vi "Process.vi"(8 "error in":errorcluster, 11 "Plugin in":refnum<class "StreamReader.lvclass">) -> (0 "error out":errorcluster, 3 "Plugin out":refnum<class "StreamReader.lvclass">)   [LabVIEW 2024, in "StreamReader.lvlib" / "StreamReader.lvclass"]
uses:
  StreamReader.lvclass
  C:/Program Files/National Instruments/LabVIEW 2024/vi.lib/FlexLogger/SDK/PluginSDK.lvlibp/PEFClasses/SDK/Plugin/Plugin.lvclass
  StreamReader.lvclass/StreamReader.ctl
  <vilib>/FlexLogger/SDK/PluginSDK.lvlibp/PEFClasses/SDK/Plugin/DataHelpers/Write 1D Wfm (DBL)_v2.vi
  <vilib>/FlexLogger/SDK/PluginSDK.lvlibp/PEFClasses/SDK/Plugin/Plugin.lvclass
  C:/Program Files/National Instruments/LabVIEW 2024/vi.lib/FlexLogger/SDK/PluginSDK.lvlibp/PEFClasses/SDK/Processing Element/Processing Element.lvclass
  C:/Users/Administrator/Documents/LabVIEW Projects/FlexLogger IO Plug-ins/StreamReader/StreamReader.lvclass
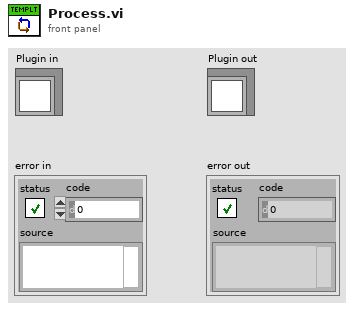
[diagram p1: front panel]
types:
  T1 = typedef "StreamReader.lvlib/StreamReader.lvclass/StreamReader Parameters.ctl" = cluster{"Reader URL":string, "Writer URL":string, "Timeout":i32, "Buffer Size":i32, "Reader endpoint":refnum<k21>, "Channel Names":string[]}
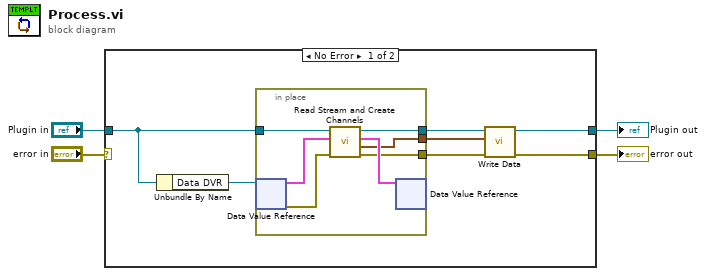
[diagram p0: block diagram]
diagram:
  n1 = case shown="No Error" "error in" {
    selector: "error in" -> [_ w19]
    tunnel: [w10 w20] -> w1
    tunnel: "Plugin in" -> [w5 w20]
    tunnel: [w11 w19] -> w2
    frame No Error {
      n2 = Unbundle By Name(w5) -> ("Data DVR"=w9:refnum<data-value>)
      n3 = in-place {
        in-place-border: w5 -> [w18]
        in-place-border: [w15] -> w8
        in-place-border: [w13] -> w7
        in-place-border: [w12] -> w6
        n4 = in-place-dvr #1(w9) -> (w17:T1, w16:errorcluster)
        n5 = call-dynamic "Read Stream and Create Channels.vi"("error in (no error)"=w16, "StreamReader Parameters in"=w17, "Plugin in"=w18) -> ("error out"=w13:errorcluster, "Array"=w12:waveform(dbl)[], "StreamReader Parameters out"=w14:T1, "Plugin out"=w15:refnum<class "StreamReader.lvclass">)  [unwired: 5 in]
        n6 = in-place-dvr #1(w14) -> ()  [unwired: 2 out]
      }
      n7 = call-poly <vilib>:"Write Data.vi"("error in (no error)"=w7, "Data"=w6, "Plugin in"=w8) -> ("error out"=w11:errorcluster, "Plugin out"=w10:refnum<class "StreamReader.lvclass">)  [unwired: 7 in]
    }
    frame Error {
    }
  }
  "error out" <- w2
  "Plugin out" <- w1
